vi "Write_file_sub_VI.vi"(11 "Output String":string) -> (1 "File Contents":string, 2 "CSV File Path":path, 3 "Current VI's path":path)   [LabVIEW 2017]
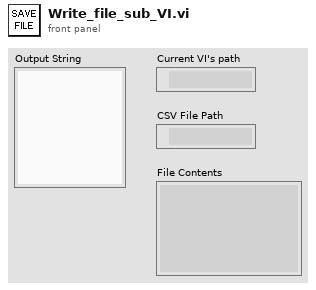
[diagram p1: front panel]
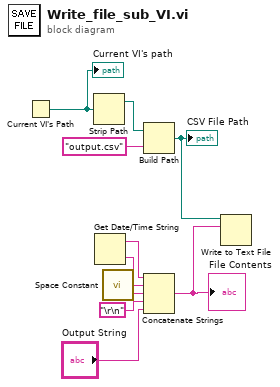
[diagram p0: block diagram]
diagram:
  n1 = Current VI's Path() -> (path=w1:path)
  "Current VI's path" <- w1
  n2 = Strip Path(path=w1) -> (stripped path=w2:path)  [unwired: 1 out]
  n3 = Get Date/Time String() -> (date string=w5:string, time string=w6:string)  [unwired: 3 in]
  n4 = call <vilib>:"Space Constant.vi"() -> ("String"=w8:string)
  n5 = Build Path(base path=w2, name or relative path="output.csv") -> (appended path=w3:path)
  "CSV File Path" <- w3
  n6 = Concatenate Strings(w5, w8, w6, "\r\n", "Output String") -> (w10:string)
  "File Contents" <- w10
  n7 = Write to Text File(file (use dialog)=w3, text=w10) -> ()  [unwired: 2 in, 3 out]
